vi "自动测试类型3统计结果.vi"   [LabVIEW 2010]
uses:
  全局量/自动测试结果.vi
  全局量/试验配置信息.vi
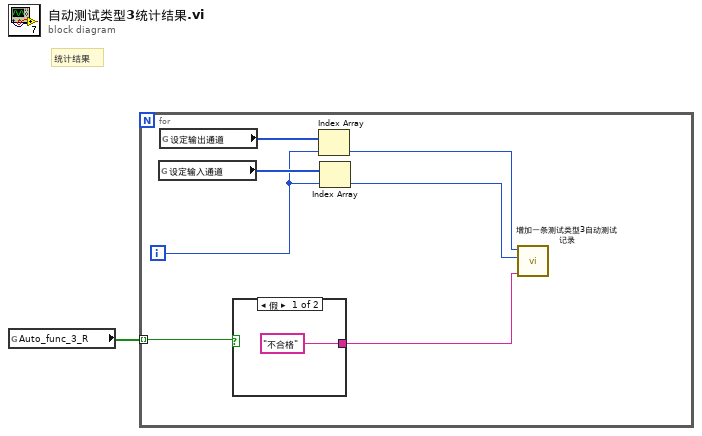
[diagram p0: block diagram]
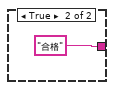
[diagram p2: hidden frame]
diagram:
  # "统计结果"
  n1 = global read "自动测试结果.vi" "Auto_func_3_R"() -> (w1:bool[])
  n2 = for {
    tunnel: w1 -> [w8] mode=indexing
    i -> [w5]
    n3 = global read "试验配置信息.vi" "设定输入通道"() -> (w6:i32[])
    n4 = global read "试验配置信息.vi" "设定输出通道"() -> (w7:i32[])
    n5 = case shown="假" w8 {
      tunnel: ["不合格" "合格"] -> w2
      frame False {
      }
      frame True {
      }
    }
    n6 = Index Array(array=w7, index=w5) -> (element=w4:i32)
    n7 = Index Array(array=w6, index=w5) -> (element=w3:i32)
    n8 = call "增加一条测试类型3自动测试记录.vi"("测试结果"=w2, "输入通道"=w3, "输出通道"=w4) -> ()  [unwired: 9 in]
  }
